vi "BMP_file_name.vi"(0 "Path_to_folder_to_save_bmp_imgs":string, 5 "Additional_text_information":string, 7 "Laser_status_ON_OFF":bool, 9 "time stamp":timestamp, 11 "Image_number":i32) -> (4 "file path":path)   [LabVIEW 2021]
panel:
  out "date/time string":string
  out "Time_ON_OFF_string":string
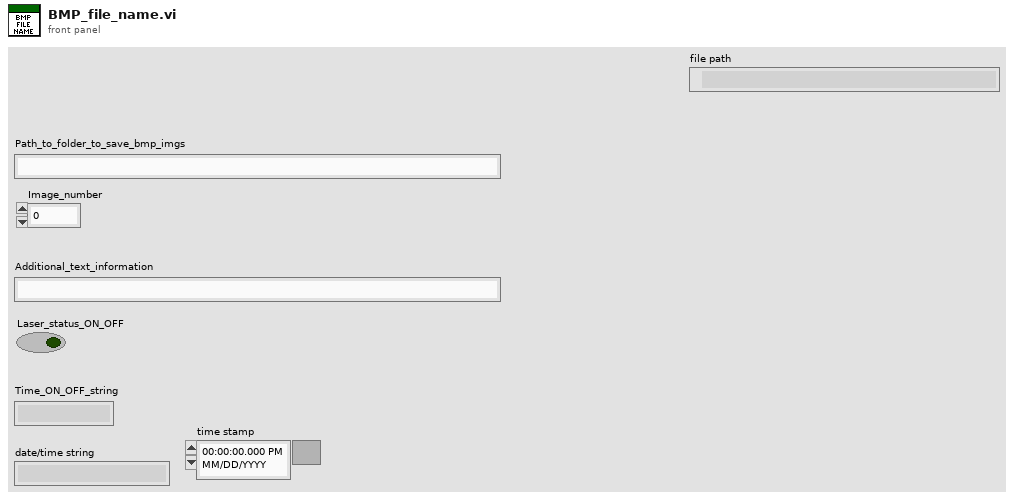
[diagram p1: front panel]
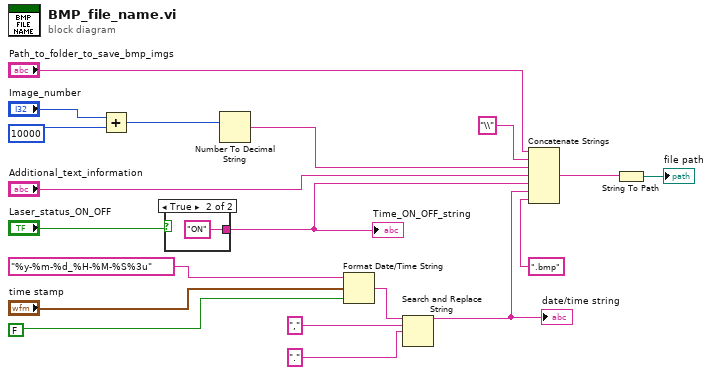
[diagram p0: block diagram]
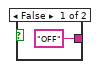
[diagram p2: hidden frame]
diagram:
  n1 = Add(x="Image_number", y=10000) -> (x+y=w3:i32)
  n2 = case shown="True" "Laser_status_ON_OFF" {
    tunnel: ["OFF" "ON"] -> w13
    frame False {
    }
    frame True {
    }
  }
  "Time_ON_OFF_string" <- w13
  n3 = Number To Decimal String(number=w3) -> (decimal integer string=w9:string)  [unwired: 1 in]
  n4 = Format Date/Time String(time format string (%c)="%y-%m-%d_%H-%M-%S%3u", seconds (now)="time stamp", UTC format=FALSE) -> (date/time string=w17:string)
  n5 = Search and Replace String(input string=w17, search string=",", replace string="." ("replace string (\"\")")) -> (result string=w12:string)  [unwired: 5 in, 3 out]
  "date/time string" <- w12
  n6 = Concatenate Strings("Path_to_folder_to_save_bmp_imgs", "\\" ("string"), w9, "Additional_text_information", w13, w12, ".bmp" ("string")) -> (w2:string)
  n7 = String To Path(string=w2) -> (path=→"file path":path)
